vi "Write Report Display.vi"(8 "error in (no error)":errorcluster, 10 "Report Display":refnum<vi>, 11 "Reports in":refnum<class "Results.lvclass">) -> (0 "error out":errorcluster, 3 "Reports out":refnum<class "Results.lvclass">)   [LabVIEW 2016, in "Result Actor.lvlib" / "Results.lvclass"]
uses:
  <userlib>/Common Components/Results/Results.lvclass
  <userlib>/Common Components/Results/Results.lvclass/Results.ctl
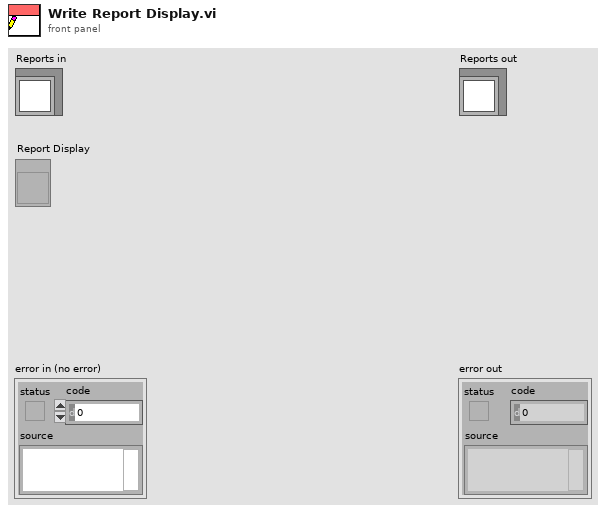
[diagram p1: front panel]
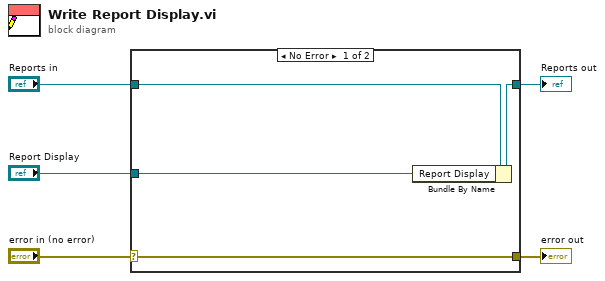
[diagram p0: block diagram]
diagram:
  n1 = case shown="No Error" "error in (no error)" {
    selector: "error in (no error)" -> [w9 w10]
    tunnel: [w9 w10] -> w4
    tunnel: [w7 w11] -> w2
    tunnel: "Reports in" -> [w8 w11]
    tunnel: "Report Display" -> [w6 _]
    frame No Error {
      n2 = Bundle By Name(cluster=w8, "Report Display"=w6) -> (w7:refnum<class "Results.lvclass">)
    }
    frame Error {
    }
  }
  "error out" <- w4
  "Reports out" <- w2
